vi "ArrayBundlesToDisplay.vi"(1 "Array":T1(array[cluster]) {"End" format="%<%.3X>T"; "Start" format="%<%.3X>T"}) -> (0 "Array 2":string[](array[string]))   [LabVIEW 2017]
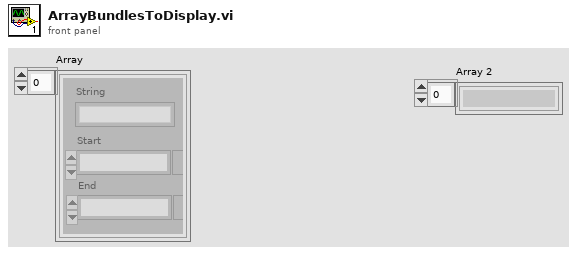
[diagram p1: front panel]
types:
  T1 = cluster{"String":string, "Start":timestamp, "End":timestamp}[]
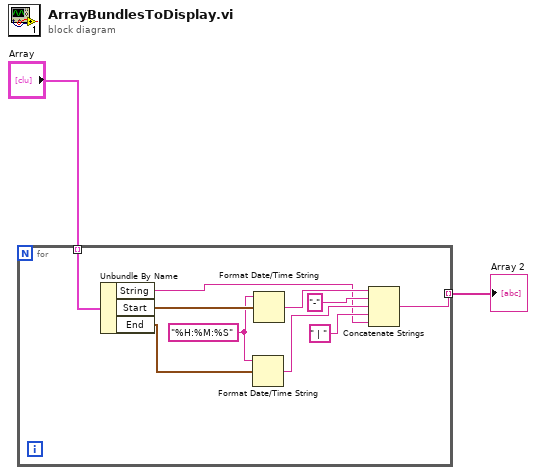
[diagram p0: block diagram]
diagram:
  n1 = for {
    tunnel: "Array" -> [w12] mode=indexing
    tunnel: [w9] -> w1 mode=indexing
    w7 = "%H:%M:%S"
    n2 = Unbundle By Name(w12) -> ("String"=w3:string, "Start"=w11:timestamp, "End"=w8:timestamp)
    n3 = Format Date/Time String(time format string (%c)=w7, seconds (now)=w8) -> (date/time string=w5:string)  [unwired: 1 in]
    n4 = Format Date/Time String(time format string (%c)=w7, seconds (now)=w11) -> (date/time string=w10:string)  [unwired: 1 in]
    n5 = Concatenate Strings(w10, "-", w5, " | ", w3) -> (w9:string)
  }
  "Array 2" <- w1
